vi "Settings User Event.vi"(8 "error in (no error)":errorcluster, 11 "Action":enum16{"Create", "Get", "Destroy"}(ring)) -> (0 "error out":errorcluster, 3 "TermCurrentSetting":refnum<user-event>)   [LabVIEW 2018]
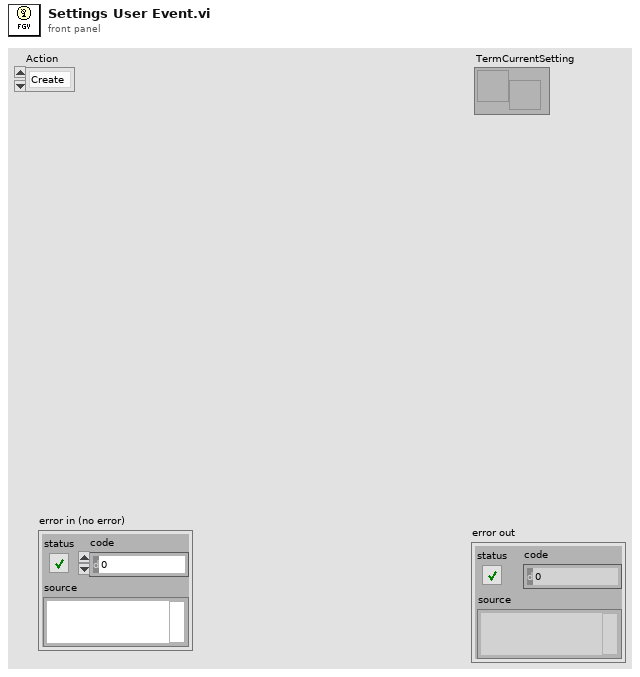
[diagram p1: front panel]
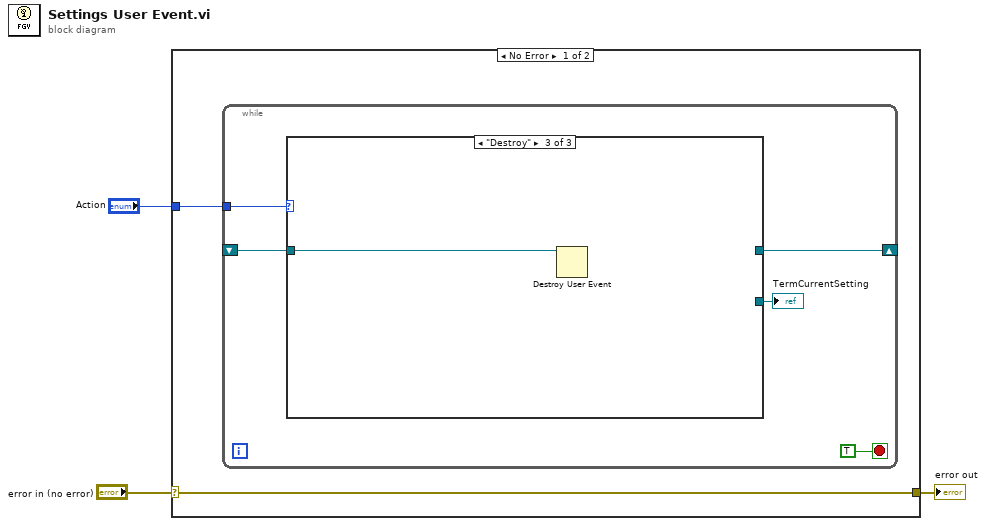
[diagram p0: block diagram]
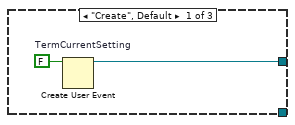
[diagram p2: hidden frame]
diagram:
  n1 = case shown="No Error" "error in (no error)" {
    selector: "error in (no error)" -> [w5 w15]
    tunnel: [w5 w15] -> w2
    tunnel: "Action" -> [w4 _]
    frame No Error {
      n2 = while {
        tunnel: w4 -> [w10]
        shift-right: [w9] -> _
        shift-left: _ -> [w8]
        stop <- TRUE stop-if-true
        n3 = case shown="\"Destroy\"" w10 {
          tunnel: [w12 w13 _] -> w9
          tunnel: w8 -> [_ w13 w14]
          tunnel: [_ w13 _] -> w7
          frame "Create", Default {
            w11 = FALSE  # TermCurrentSetting
            n4 = Create User Event(user event datatype=w11) -> (user event=w12:refnum<user-event>)  [unwired: 1 in, 1 out]
          }
          frame "Get" {
          }
          frame "Destroy" {
            n5 = Destroy User Event(user event=w14) -> ()  [unwired: 1 in, 1 out]
          }
        }
        "TermCurrentSetting" <- w7
      }
    }
    frame Error {
    }
  }
  "error out" <- w2
